vi "Shutdown Sequence.vi"(0 "CANOpen Session":refnum<k20>, 1 "CAN Session":T1, 7 "error in (no error)":errorcluster, 10 "Update Motors Notifier":refnum<notifier>, 11 "Right motor Clustered SDO":T2, 12 "Shutdown Notifier":refnum<notifier>, 13 "Left motor Clustered SDO":T2, 14 "Emergency Turn Off Notifier":refnum<notifier>, 16 "Error Queue":refnum<queue>) -> (27 "error out":errorcluster)   [LabVIEW 2016]
uses:
  RT/Clustered SDO.ctl
  Program Files (x86)/National Instruments/LabVIEW 2016/examples/robotics/EPOS2 CANOpen Driver/Low Level VIs/Typedefs/CAN Refnum.ctl
  Program Files (x86)/National Instruments/LabVIEW 2016/examples/robotics/EPOS2 CANOpen Driver/Low Level VIs/Typedefs/CAN Session Pointer.ctl
  Program Files (x86)/National Instruments/LabVIEW 2016/examples/robotics/EPOS2 CANOpen Driver/Low Level VIs/Typedefs/CAN Communication References.ctl
  Program Files (x86)/National Instruments/LabVIEW 2016/examples/robotics/EPOS2 CANOpen Driver/Low Level VIs/Typedefs/kill process notifier array.ctl
  Program Files (x86)/National Instruments/LabVIEW 2016/examples/robotics/EPOS2 CANOpen Driver/Low Level VIs/Typedefs/Write Queue.ctl
  Program Files (x86)/National Instruments/LabVIEW 2016/examples/robotics/EPOS2 CANOpen Driver/Low Level VIs/Typedefs/FPGA CAN Frame Cluster.ctl
  <vilib>/CANopenLib/CANOPEN.llb/CANopen SDO Close.vi
  <vilib>/CANopenLib/CANOPEN.llb/CANopen Interface Close.vi
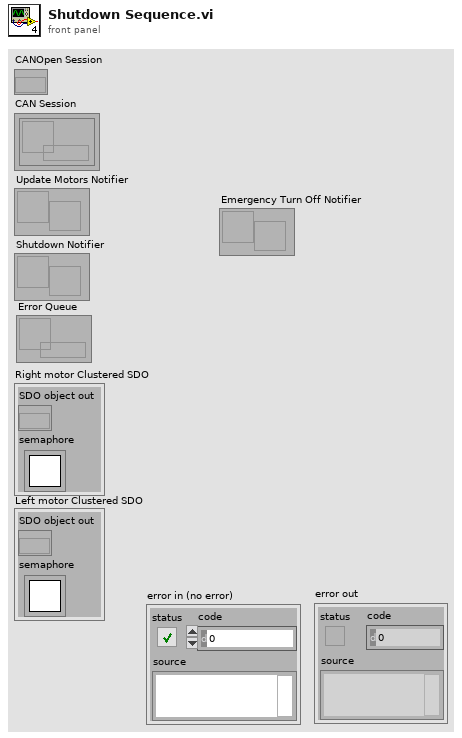
[diagram p1: front panel]
types:
  T1 = typedef "CAN Refnum.ctl" = refnum<k1>
  T2 = typedef "Clustered SDO.ctl" = cluster{"SDO object out":refnum<k20>, "semaphore":T3}
  T3 = typedef "Semaphore RefNum" = refnum<k1>
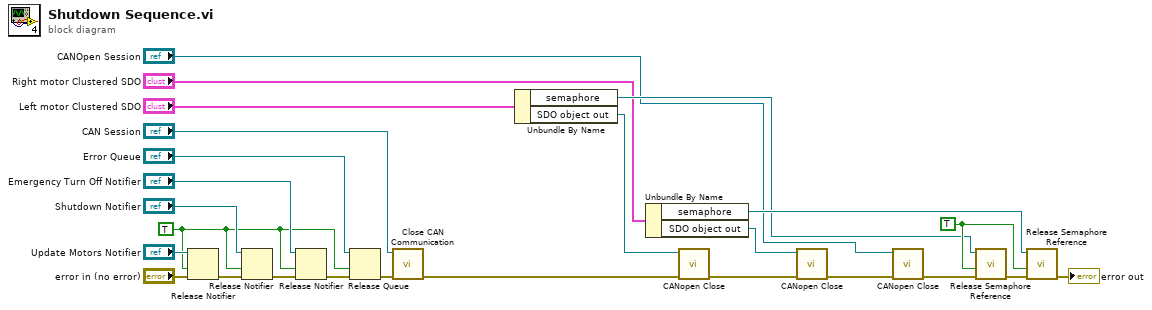
[diagram p0: block diagram]
diagram:
  w22 = TRUE ("force destroy? (F)")
  w5 = TRUE
  n1 = Release Notifier(notifier="Update Motors Notifier", force destroy? (F)=w5, error in (no error)="error in (no error)") -> (error out=w4:errorcluster)  [unwired: 2 out]
  n2 = Release Notifier(notifier="Shutdown Notifier", force destroy? (F)=w5, error in (no error)=w4) -> (error out=w3:errorcluster)  [unwired: 2 out]
  n3 = Release Notifier(notifier="Emergency Turn Off Notifier", force destroy? (F)=w5, error in (no error)=w3) -> (error out=w2:errorcluster)  [unwired: 2 out]
  n4 = Release Queue(queue="Error Queue", force destroy? (F)=w5, error in (no error)=w2) -> (error out=w1:errorcluster)  [unwired: 2 out]
  n5 = call "Close CAN Communication.vi"("error in"=w1, "CAN Session"="CAN Session") -> ("error out"=w20:errorcluster)  [unwired: 9 in]
  n6 = Unbundle By Name("Left motor Clustered SDO") -> ("semaphore"=w17:T3, "SDO object out"=w18:refnum<k20>)
  n7 = Unbundle By Name("Right motor Clustered SDO") -> ("semaphore"=w21:T3, "SDO object out"=w16:refnum<k20>)
  n8 = call-poly <vilib>:"CANopen Close.vi"("error in (no error)"=w20, "SDO object in"=w18) -> ("error out"=w19:errorcluster)  [unwired: 9 in]
  n9 = call-poly <vilib>:"CANopen Close.vi"("error in (no error)"=w19, "SDO object in"=w16) -> ("error out"=w25:errorcluster)  [unwired: 9 in]
  n10 = call-poly <vilib>:"CANopen Close.vi"("error in (no error)"=w25, "interface object in"="CANOpen Session") -> ("error out"=w23:errorcluster)  [unwired: 9 in]
  n11 = call <vilib>:"Release Semaphore Reference.vi"("error in (no error)"=w23, "force destroy? (F)"=w22, "semaphore"=w17) -> ("error out"=w24:errorcluster)  [unwired: 7 in, 1 out]
  n12 = call <vilib>:"Release Semaphore Reference.vi"("error in (no error)"=w24, "force destroy? (F)"=w22, "semaphore"=w21) -> ("error out"=→"error out":errorcluster)  [unwired: 7 in, 1 out]
